vi "Counts Since Last Reset.vi"(6 "Reset (F)":bool, 7 "Error In":errorcluster) -> (2 "counter":u32, 3 "Error Out":errorcluster)   [LabVIEW 2019, in "Instrument.lvlib" / "Instrument.lvclass"]
doc: "Returns the amount of time in milliseconds since the last time the VI was reset. This VI is non-reentrant.\n\nAuthored by Brandon D. Steele\nsupport@mooregoodideas.com\nwww.mooregoodideas.com\n\nCopyright (c) 2010, Moore Good Ideas, Inc.\n\nAll rights reserved.\n\nRedistribution and use in source and binary forms, with or without modification, are permitted provided that the following conditions are met:\n\n * Redistributions of source code must retain the above copyright notice, this list of conditions and the following disclaimer.\n * Redistributions in binary form must reproduce the above copyright notice, this list of conditions and the following disclaimer in the documentation and/or other materials provided with the distribution.\n * Neither the name of Moore Good Ideas, Inc. nor the names of its contributors may be used to endorse or promote products derived from this software without specific prior written permission.\n\nTHIS SOFTWARE IS PROVIDED BY THE COPYRIGHT HOLDERS AND CONTRIBUTORS \"AS IS\" AND ANY EXPRESS OR IMPLIED WARRANTIES, INCLUDING, BUT NOT LIMITED TO, THE IMPLIED WARRANTIES OF MERCHANTABILITY AND FITNESS FOR A PARTICULAR PURPOSE ARE DISCLAIMED. IN NO EVENT SHALL THE COPYRIGHT OWNER OR CONTRIBUTORS BE LIABLE FOR ANY DIRECT, INDIRECT, INCIDENTAL, SPECIAL, EXEMPLARY, OR CONSEQUENTIAL DAMAGES (INCLUDING, BUT NOT LIMITED TO, PROCUREMENT OF SUBSTITUTE GOODS OR SERVICES; LOSS OF USE, DATA, OR PROFITS; OR BUSINESS INTERRUPTION) HOWEVER CAUSED AND ON ANY THEORY OF LIABILITY, WHETHER IN CONTRACT, STRICT LIABILITY, OR TORT (INCLUDING NEGLIGENCE OR OTHERWISE) ARISING IN ANY WAY OUT OF THE USE OF THIS SOFTWARE, EVEN IF ADVISED OF THE POSSIBILITY OF SUCH DAMAGE."
uses:
  Instrument.lvclass
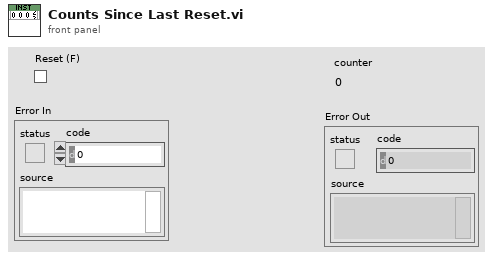
[diagram p1: front panel]
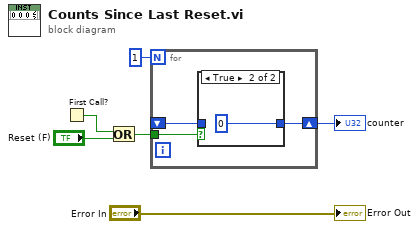
[diagram p0: block diagram]
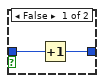
[diagram p2: hidden frame]
diagram:
  n1 = First Call?() -> (First Call?: T/F=w2:bool)
  n2 = Or(x=w2, y="Reset (F)") -> (x .or. y?=w1:bool)
  n3 = for {
    N: 1 -> [_]
    shift-right: [w9] -> w4
    shift-left: _ -> [w8]
    tunnel: w1 -> [w7]
    n4 = case shown="True" w7 {
      tunnel: [w11 u32 0 ("millisecond timer value")] -> w9
      tunnel: w8 -> [w10 _]
      frame False {
        n5 = Increment(x=w10) -> (x+1=w11:u32)
      }
      frame True {
      }
    }
  }
  "counter" <- w4
  "Error Out" <- "Error In"
